vi "File-Suffix.vi"(1 "Substring":string, 2 "String 2":string) -> (0 "String":string)   [LabVIEW 2013]
panel:
  # "Copyright Americo A. Migliaccio (c) 2002 All Rights Reserved by Author"
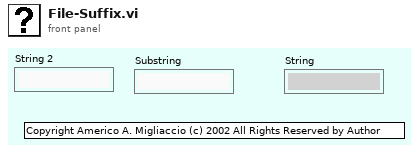
[diagram p1: front panel]
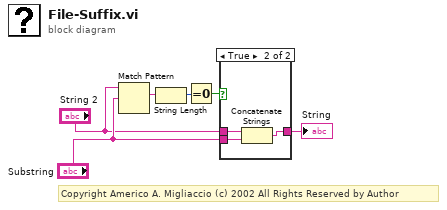
[diagram p0: block diagram]
diagram:
  # "Copyright Americo A. Migliaccio (c) 2002 All Rights Reserved by Author"
  n1 = Match Pattern(string="String 2", regular expression="Substring") -> (match substring=w1:string)  [unwired: 1 in, 3 out]
  n2 = String Length(string=w1) -> (length=w2:i32)
  n3 = Equal To 0?(x=w2) -> (x = 0?=w3:bool)
  n4 = case shown="True" w3 {
    tunnel: "String 2" -> [w7 w10]
    tunnel: "Substring" -> [_ w9]
    tunnel: [w7 w8] -> w6
    frame False {
    }
    frame True {
      n5 = Concatenate Strings(w10, w9) -> (w8:string)
    }
  }
  "String" <- w6
